vi "Demo_Static.vi"() -> ()   [LabVIEW 2012]
uses:
  WaveGraphX.xctl
  <vilib>/measure/NI_MABase.lvlib
panel:
  out "波形图":dbl[][](graph)
  in  "停止":bool
  out "WaveGraphX":dbl[][](xcontrol)
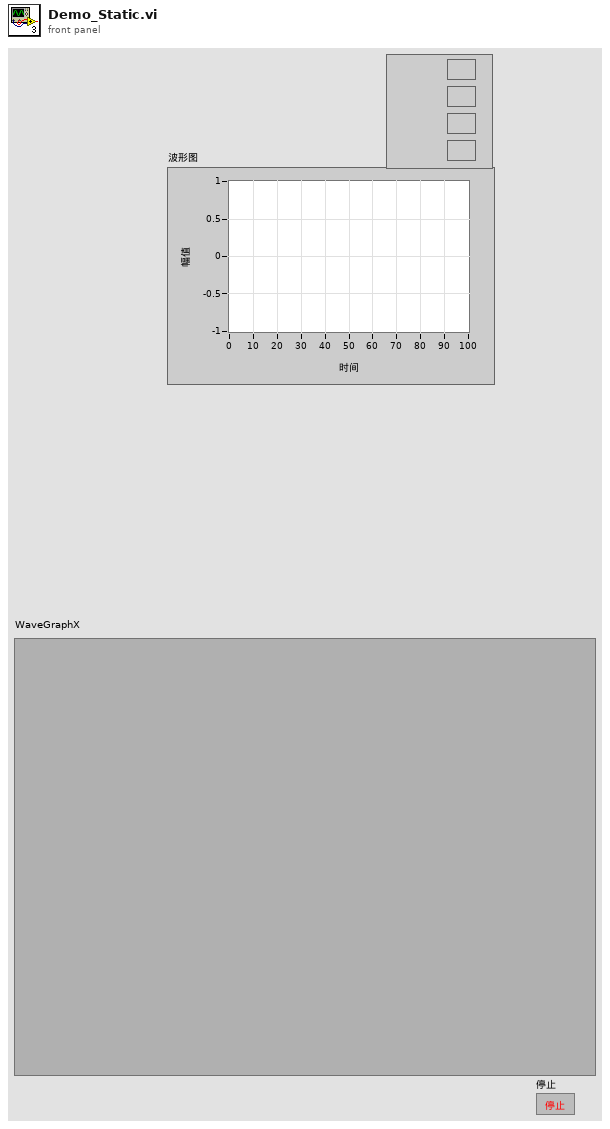
[diagram p1: front panel]
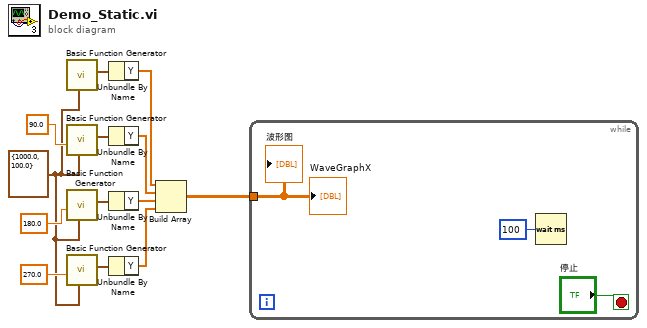
[diagram p0: block diagram]
diagram:
  w5 = cluster{"Fs":dbl, "#s":dbl} {"Fs"=1000.0, "#s"=100.0} ("sampling info")
  n1 = call <vilib>:"Basic Function Generator.vi"("sampling info"=w5) -> ("signal out"=w13:waveform(dbl))  [unwired: 8 in, 2 out]
  n2 = call <vilib>:"Basic Function Generator.vi"("sampling info"=w5, "phase"=90.0) -> ("signal out"=w9:waveform(dbl))  [unwired: 7 in, 2 out]
  n3 = call <vilib>:"Basic Function Generator.vi"("sampling info"=w5, "phase"=180.0) -> ("signal out"=w3:waveform(dbl))  [unwired: 7 in, 2 out]
  n4 = call <vilib>:"Basic Function Generator.vi"("sampling info"=w5, "phase"=270.0) -> ("signal out"=w4:waveform(dbl))  [unwired: 7 in, 2 out]
  n5 = Unbundle By Name(w13) -> ("Y"=w12:dbl[])
  n6 = Unbundle By Name(w9) -> ("Y"=w8:dbl[])
  n7 = Unbundle By Name(w3) -> ("Y"=w2:dbl[])
  n8 = Unbundle By Name(w4) -> ("Y"=w1:dbl[])
  n9 = Build Array(w12, w8, w2, w1) -> (w11:dbl[][])
  n10 = while {
    tunnel: w11 -> [w14]
    stop <- "停止" stop-if-true
    n11 = Wait (ms)(milliseconds to wait=u32 100 ("等待时间（毫秒）")) -> ()  [unwired: 1 out]
    "WaveGraphX" <- w14
    "波形图" <- w14
  }
